vi "write single register.vi"(8 "error in (no error)":errorcluster, 9 "register to write":u16 format="%.0x", 10 "address":u16 format="%.0x", 11 "Stepper in":refnum<class "Stepper.lvclass">) -> (0 "error out":errorcluster, 3 "Stepper out":refnum<class "Stepper.lvclass">)   [LabVIEW 2025, in "Motor.lvlib" / "Stepper.lvclass"]
uses:
  Stepper.lvclass
  Stepper.lvclass/Stepper.ctl
  <vilib>/NI/Modbus Library/API/Master/Modbus Master.lvclass
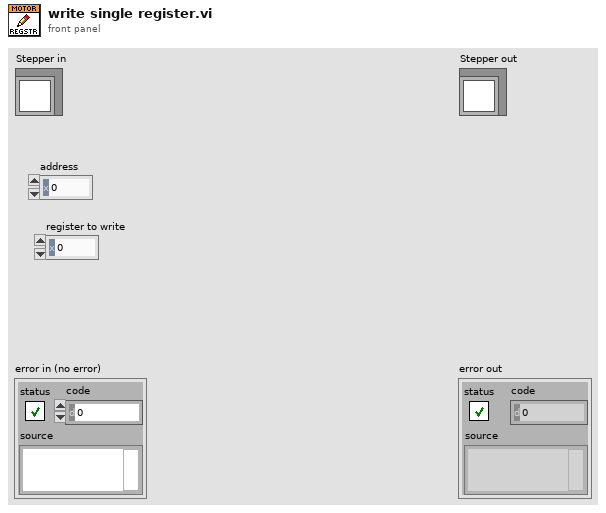
[diagram p1: front panel]
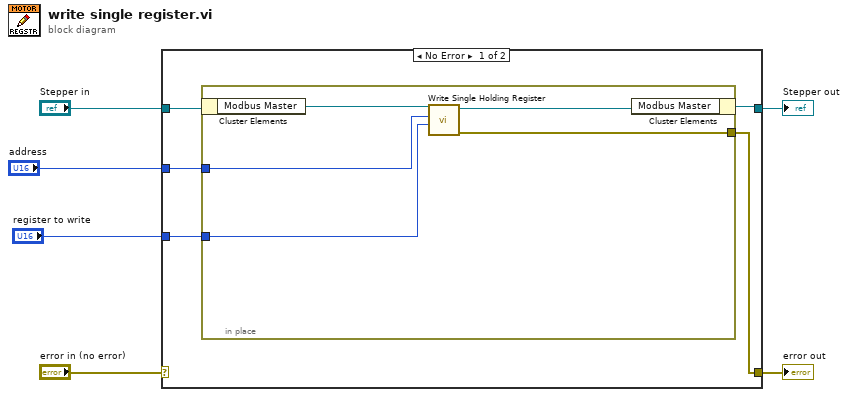
[diagram p0: block diagram]
diagram:
  n1 = case shown="No Error" "error in (no error)" {
    selector: "error in (no error)" -> [_ w18]
    tunnel: [w7 w18] -> w5
    tunnel: [w10 w17] -> w3
    tunnel: "Stepper in" -> [w11 w17]
    tunnel: "address" -> [w9 _]
    tunnel: "register to write" -> [w8 _]
    frame No Error {
      n2 = in-place {
        in-place-border: w9 -> [w14]
        in-place-border: w8 -> [w13]
        in-place-border: [w12] -> w7
        n3 = in-place-cluster #1(w11) -> ("Modbus Master"=w16:refnum<class "Modbus Master.lvclass">)
        n4 = call-dynamic "Write Single Holding Register.vi"("register to write"=w13, "address"=w14, "Modbus master in"=w16) -> ("error out"=w12:errorcluster, "Modbus master out"=w15:refnum<class "Modbus Master.lvclass">)  [unwired: 7 in]
        n5 = in-place-cluster #1("Modbus Master"=w15) -> (w10:refnum<class "Stepper.lvclass">)
      }
    }
    frame Error {
    }
  }
  "error out" <- w5
  "Stepper out" <- w3
